vi "lab4_sim_cp_ofdm_transceiver.vi"() -> ()   [LabVIEW 2014]
uses:
  <vilib>/addons/Modulation/Digital/General/MT Generate Bits (Galois, PN Order).vi
  <vilib>/Analysis/2dsp.llb/Inverse Complex FFT.vi
  <vilib>/Analysis/2dsp.llb/Complex FFT.vi
  <vilib>/Analysis/5stat.llb/RMS (DBL).vi
  <vilib>/addons/Modulation/Digital/Support/Common/Validators/mod_Generate Bits Validate.vi
  <vilib>/addons/Modulation/Analog/support/mod_Set Error Source.vi
  <vilib>/addons/Modulation/Digital/General/MT Generate QAM System Parameters(M).vi
  <vilib>/addons/Modulation/Digital/General/subVIs/mod_Generate Bits PN Sequence.vi
  <vilib>/addons/Modulation/Digital/General/MT Map Bits to QAM Symbols.vi
  <vilib>/gmath/statdist.llb/Normal Random.vi
  <vilib>/addons/Modulation/Digital/General/MT Map QAM Symbols to Bits.vi
  <vilib>/Analysis/NI_AALPro.lvlib
  <vilib>/addons/Modulation/niDMT.lvlib
  <vilib>/gmath/NI_Gmath.lvlib
panel:
  out "pilot channel gain":dbl[](graph)
  out "pilot channel gain":dbl[](graph)
  out "PAPR":dbl
  out "Error bits":i32
  out "Bit compare":bool[](array[boolean])
  out "BER":dbl
  in  "millisecond multiple":u32=20
  out "output bit stream 2":i8[](array[numeric]) caption="Transmit output bit stream"
  out "output bit stream":i8[](array[numeric]) caption="Received output bit stream"
  in  "M-QAM (16)":i32=16
  out "Transmit FFT (Magnitude)":dbl[](graph)
  out "Receiver FFT (Magnitude)":dbl[](graph)
  out "RX constellation":cdb[](graph)
  in  "pilot carrier":i32=32
  in  "message carrier":i32=120
  out "eb/n0 (dB)":dbl=38.96307662438871
  in  "Symbol energy es/n0(db)":dbl=50.0 format="%#_13g"
  in  "stop":bool
  in  "cyclic prefix":i32=64
  in  "FFT size":i32=256
  in  "ofdm symbols":i32=10
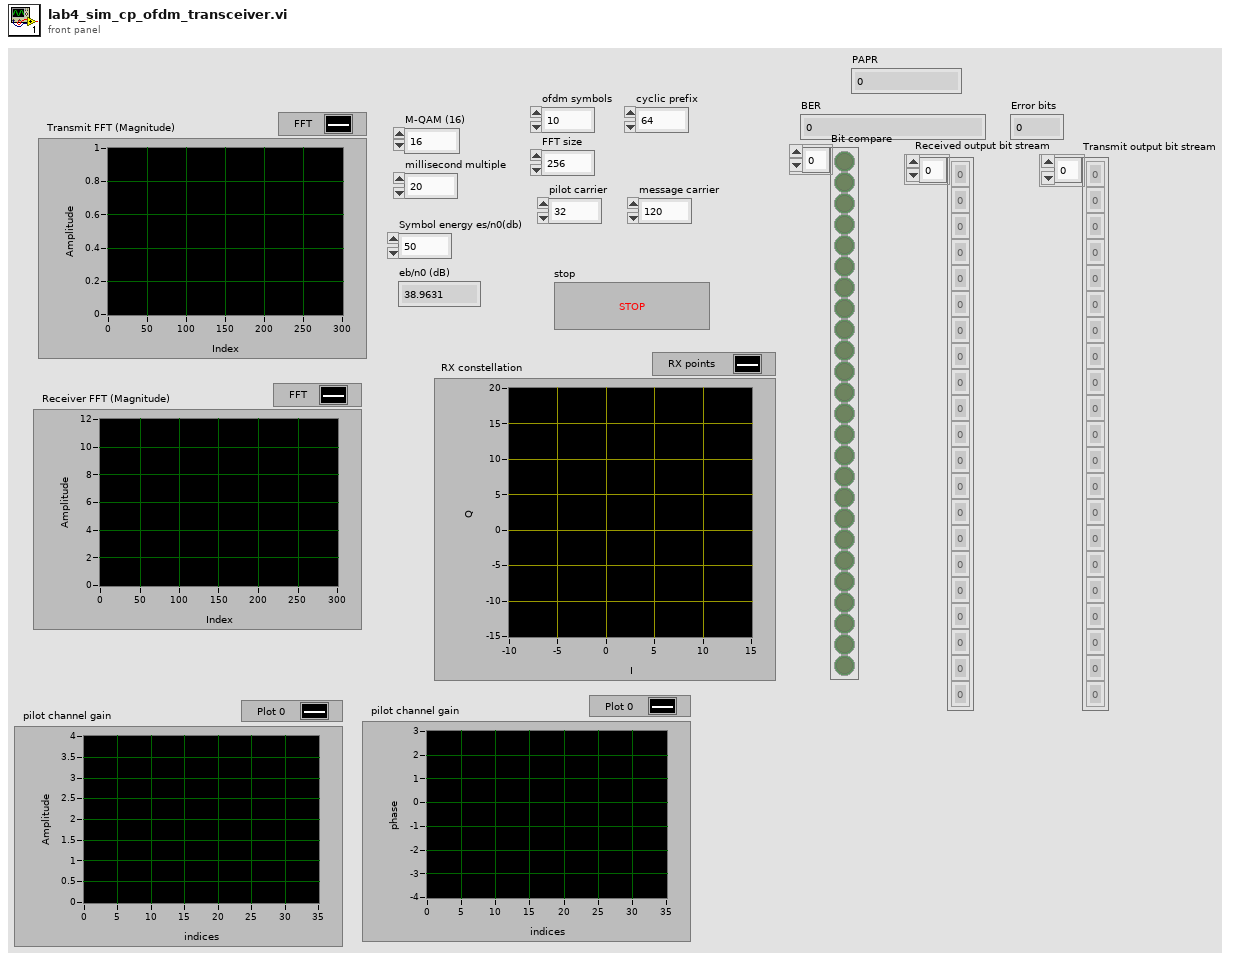
[diagram p1: front panel]
types:
  T1 = cluster{"samples per symbol (16)":i32, "symbol map":cdb[]}
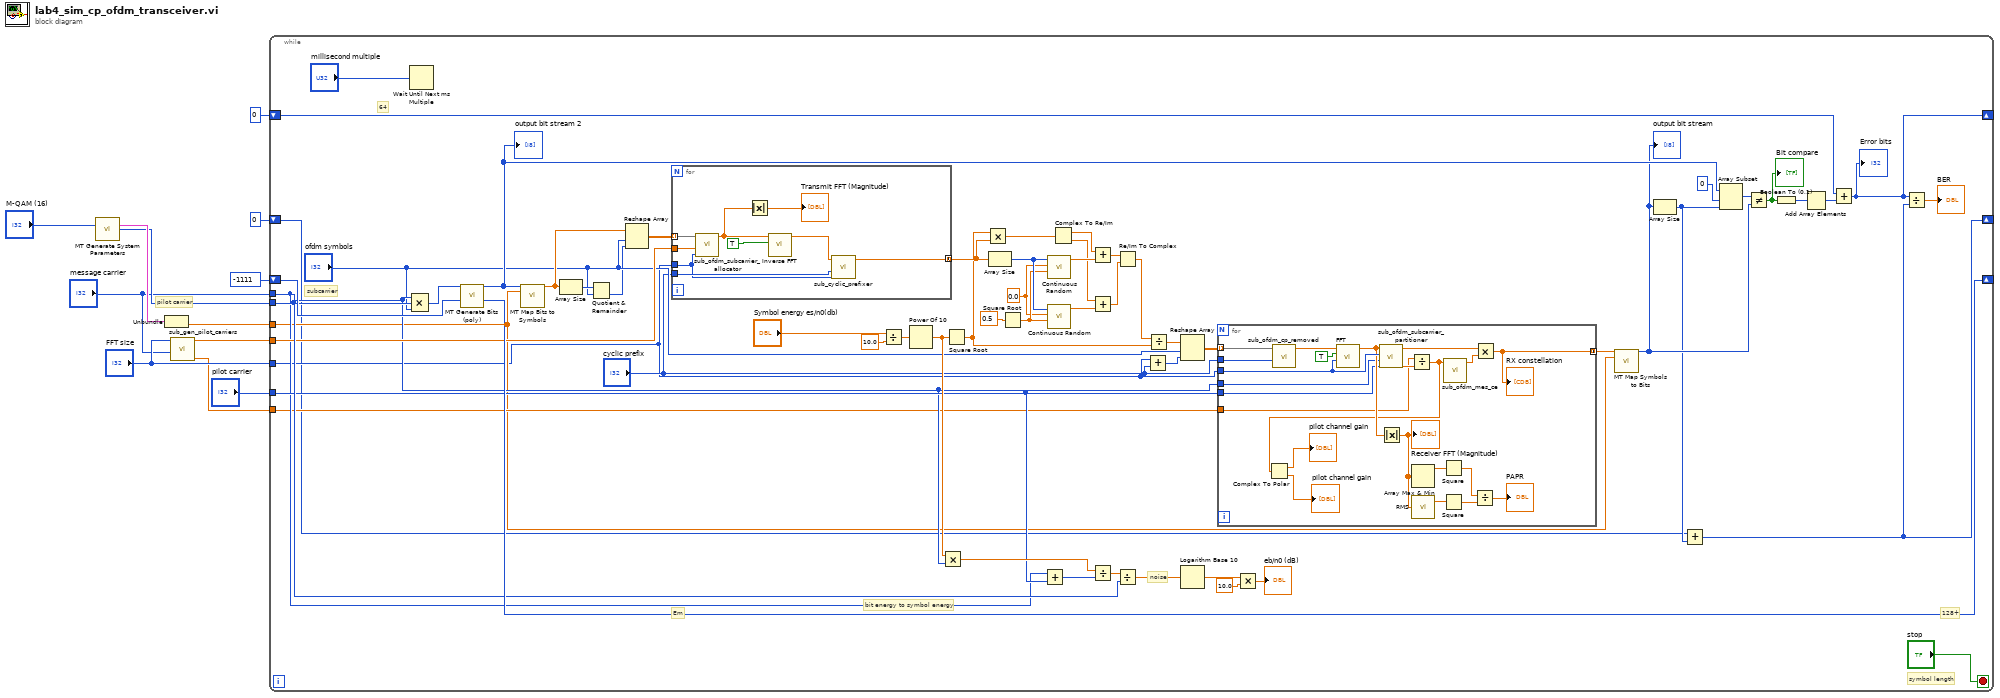
[diagram p0: block diagram]
diagram:
  # "pilot carrier"
  n1 = call-poly <vilib>:"MT Generate System Parameters.vi"("M-QAM (16)"="M-QAM (16)") -> ("QAM system parameters"=w9:T1, "bits per symbol"=w7:i32)  [unwired: 12 in, 1 out]
  n2 = Unbundle(w9) -> ("symbol map"=w8:cdb[])  [unwired: 1 out]
  n3 = call "sub_gen_pilot_carriers.vi"("message carrier"="message carrier", "FFT size"="FFT size") -> ("RX pilot carriers"=w2:cdb[], "TX pilot carriers"=w1:cdb[])  [unwired: 8 in]
  n4 = while {
    tunnel: w7 -> [w58]
    shift-right: [w71] -> _
    shift-left: -1111 ("seed out") -> [w72]
    tunnel: w1 -> [w54]
    tunnel: "pilot carrier" -> [w52]
    tunnel: "message carrier" -> [w51]
    tunnel: "FFT size" -> [w35]
    tunnel: w2 -> [w50]
    tunnel: w8 -> [w49]
    shift-right: [w17] -> _
    shift-left: 0 -> [w20]
    shift-right: [w16] -> _
    shift-left: 0 -> [w18]
    stop <- "stop" stop-if-true
    w13 = 0.0 ("mean")
    # "symbol length"
    # "bit energy to symbol energy"
    # "noise"
    # "128+"
    # "subcarrier"
    # "Em"
    # "64"
    n5 = Wait Until Next ms Multiple(millisecond multiple="millisecond multiple") -> ()  [unwired: 1 out]
    n6 = Compound Arithmetic op=MULTIPLY(w51, w58, "ofdm symbols") -> (w46:i32)
    n7 = call-poly <vilib>:"MT Generate Bits (poly).vi"("total bits (128)"=w46, "seed in (0xD6BF7DF2)"=w72) -> ("output bit stream"=w44:i8[], "seed out"=w71:i32)  [unwired: 11 in, 1 out]
    "output bit stream 2" <- w44
    n8 = call-poly <vilib>:"MT Map Bits to Symbols.vi"("input bit stream"=w44, "symbol map"=w49) -> ("symbols"=w56:cdb[])  [unwired: 12 in, 1 out]
    n9 = Array Size(array=w56) -> (size(s)=w70:i32)
    n10 = Quotient & Remainder(x=w70, y="ofdm symbols") -> (floor(x/y)=w38:i32)  [unwired: 1 out]
    n11 = Reshape Array(w56, "ofdm symbols", w38) -> (w55:cdb[][])
    n12 = for {
      tunnel: w55 -> [w103] mode=indexing
      tunnel: w54 -> [w102]
      tunnel: w35 -> [w98]
      tunnel: "cyclic prefix" -> [w99]
      tunnel: [w97] -> w32 mode=concatenating
      n13 = call "sub_ofdm_subcarrier_allocator.vi"("fft size"=w98, "pilot symbol"=w102, "message symbol"=w103) -> ("OFDM symbol"=w96:cdb[])  [unwired: 8 in]
      n14 = Absolute Value(x=w96) -> (abs(x)=→"Transmit FFT (Magnitude)":dbl[])
      n15 = call-poly <vilib>:"Inverse FFT.vi"("shift?"=TRUE, "FFT {X}"=w96) -> ("X"=w100:cdb[])  [unwired: 8 in, 1 out]
      n16 = call "sub_cyclic_prefixer.vi"("FFT size"=w98, "CP length"=w99, "time_samples"=w100) -> ("cp ofdm symbol"=w97:cdb[])  [unwired: 8 in]
    }
    n17 = Divide(x="Symbol energy es/n0(db)", y=10.0) -> (x/y=w65:dbl)
    n18 = Power Of 10(x=w65) -> (10^x=w61:dbl)
    n19 = Multiply(x=w61, y=w51) -> (x*y=w60:dbl)
    n20 = Square Root(x=w61) -> (sqrt(x)=w23:dbl)
    n21 = Multiply(x=w23, y=w32) -> (x*y=w33:cdb[])
    n22 = Array Size(array=w32) -> (size(s)=w31:i32)
    n23 = Square Root(x=0.5 ("std")) -> (sqrt(x)=w14:dbl)
    n24 = Add(x=w51, y=w52) -> (x+y=w53:i32)
    n25 = call-poly <vilib>:"Continuous Random.vi"("std"=w14, "mean"=w13, "samples"=w31) -> ("normal random data"=w29:dbl[])  [unwired: 7 in, 1 out]
    n26 = call-poly <vilib>:"Continuous Random.vi"("std"=w14, "mean"=w13, "samples"=w31) -> ("normal random data"=w27:dbl[])  [unwired: 7 in, 1 out]
    n27 = Complex To Re/Im(x + iy=w33) -> (x=w30:dbl[], y=w28:dbl[])
    n28 = Add(x=w30, y=w29) -> (x+y=w26:dbl[])
    n29 = Add(x=w28, y=w27) -> (x+y=w25:dbl[])
    n30 = Divide(x=w60, y=w53) -> (x/y=w59:dbl)
    n31 = Re/Im To Complex(1:w25, 2:w26) -> (0:w24:cdb[])
    n32 = Divide(x=w59, y=w58) -> (x/y=w57:dbl)
    n33 = Add(x=w35, y="cyclic prefix") -> (x+y=w34:i32)
    n34 = Divide(x=w24, y=w23) -> (x/y=w22:cdb[])
    n35 = Reshape Array(w22, "ofdm symbols", w34) -> (w37:cdb[][])
    n36 = Logarithm Base 10(1:w57) -> (0:w64:dbl)
    n37 = for {
      tunnel: w37 -> [w94] mode=indexing
      tunnel: "cyclic prefix" -> [w93]
      tunnel: w35 -> [w90]
      tunnel: [w88] -> w40 mode=concatenating
      tunnel: w51 -> [w86]
      tunnel: w52 -> [w85]
      tunnel: w50 -> [w82]
      n38 = call "sub_ofdm_cp_removed.vi"("CP length"=w93, "time ofdm symbol"=w94) -> ("cp removed ofdm symbol"=w91:cdb[])  [unwired: 9 in]
      n39 = call-poly <vilib>:"FFT.vi"("FFT size"=w90, "shift?"=TRUE, "X"=w91) -> ("FFT {X}"=w87:cdb[])  [unwired: 7 in, 1 out]
      n40 = call "sub_ofdm_subcarrier_partitioner.vi"("pilot carrier"=w85, "message carrier"=w86, "FFT size"=w90, "received symbol"=w87) -> ("pilot subcarriers"=w89:cdb[], "message subcarriers"=w83:cdb[])  [unwired: 6 in]
      n41 = Absolute Value(x=w87) -> (abs(x)=w81:dbl[])
      "Receiver FFT (Magnitude)" <- w81
      n42 = Divide(x=w82, y=w89) -> (x/y=w75:cdb[])
      n43 = Complex To Polar(r * e^(i*theta)=w75) -> (r=→"pilot channel gain":dbl[], theta=→"pilot channel gain":dbl[])
      n44 = Array Max & Min(array=w81) -> (max value=w80:dbl)  [unwired: 3 out]
      n45 = call-poly <vilib>:"RMS.vi"("X"=w81) -> ("rms value"=w79:dbl)  [unwired: 1 out]
      n46 = Square(x=w80) -> (x^2=w78:dbl)
      n47 = Square(x=w79) -> (x^2=w77:dbl)
      n48 = call "sub_ofdm_mes_ce.vi"("ZF channel estimates"=w75) -> ("interpolated mes carrier CE"=w84:cdb[])  [unwired: 10 in]
      n49 = Divide(x=w78, y=w77) -> (x/y=→"PAPR":dbl)
      n50 = Multiply(x=w83, y=w84) -> (x*y=w88:cdb[])
      "RX constellation" <- w88
    }
    n51 = Multiply(x=w64, y=10.0) -> (x*y=→"eb/n0 (dB)":dbl)
    n52 = call-poly <vilib>:"MT Map Symbols to Bits.vi"("symbols"=w40, "symbol map"=w49) -> ("output bit stream"=w43:i8[])  [unwired: 12 in, 1 out]
    "output bit stream" <- w43
    n53 = Array Size(array=w43) -> (size(s)=w19:i32)
    n54 = Add(x=w18, y=w19) -> (x+y=w16:i32)
    n55 = Array Subset(array=w44, index=0, length=w19) -> (w41:i8[])
    n56 = Not Equal?(x=w41, y=w43) -> (x != y?=w48:bool[])
    "Bit compare" <- w48
    n57 = Boolean To (0,1)(Boolean=w48) -> (0, 1=w47:i16[])
    n58 = Add Array Elements(numeric array=w47) -> (sum=w21:i16)
    n59 = Add(x=w20, y=w21) -> (x+y=w17:i32)
    "Error bits" <- w17
    n60 = Divide(x=w17, y=w16) -> (x/y=→"BER":dbl)
  }
